vi "INIT-Settings_SERVER.vi"(7 "error in (no error)":errorcluster, 10 "Control.lvclass":refnum<class "Control-Server.lvclass">) -> (0 "error out":errorcluster, 3 "Control class out":refnum<class "Control-Server.lvclass">)   [LabVIEW 2015]
uses:
  Classes/Control/Control-Server/Control-Server.lvclass
  Classes/Config/config_names_def.ctl
  Classes/Config/Config.lvclass
  globalVarII.vi
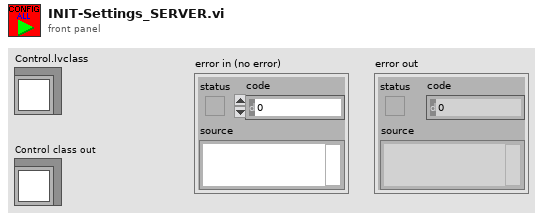
[diagram p1: front panel]
types:
  T1 = typedef "Config.lvclass/config_names_def.ctl" = string
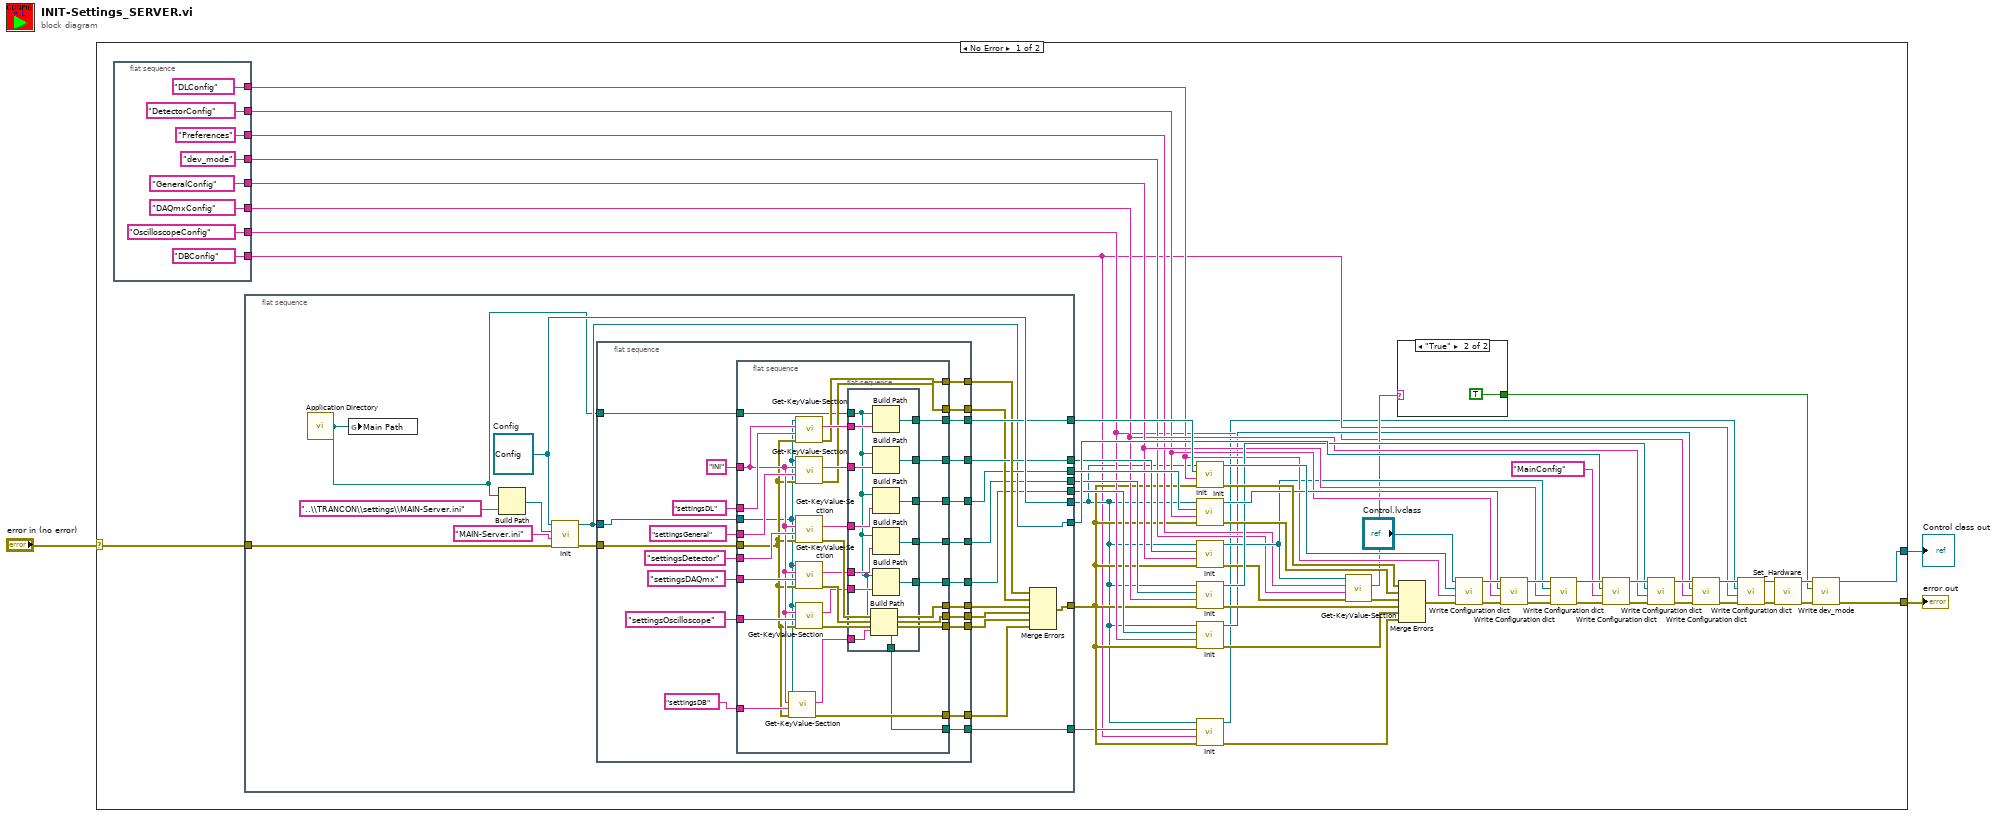
[diagram p0: block diagram]
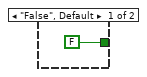
[diagram p2: hidden frame]
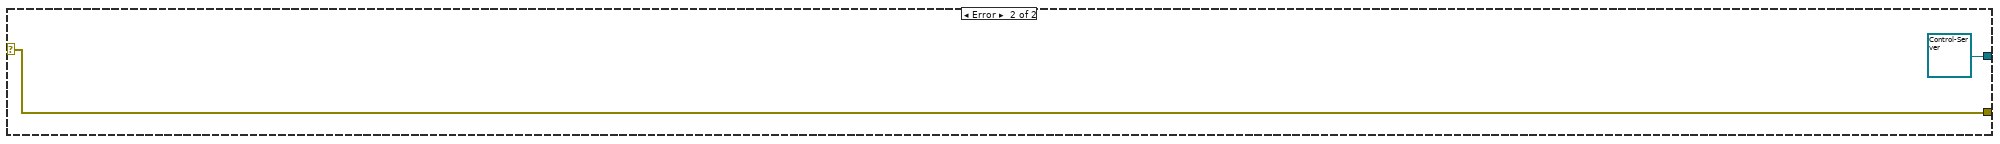
[diagram p3: hidden frame]
diagram:
  n1 = case shown="No Error" "error in (no error)" {
    selector: "error in (no error)" -> [w54 w153]
    tunnel: [w20 w153] -> w3
    tunnel: [w21 refnum<class "Control-Server.lvclass"> refnum ("Control.lvclass")] -> w1
    frame No Error {
      n2 = flat-sequence {
        tunnel: [T1 "GeneralConfig" ("Combo Box")] -> w35
        tunnel: [T1 "DAQmxConfig" ("Combo Box")] -> w34
        tunnel: [T1 "DetectorConfig" ("Combo Box")] -> w33
        tunnel: [T1 "DLConfig" ("Combo Box")] -> w32
        tunnel: ["Preferences" ("Section")] -> w25
        tunnel: ["dev_mode" ("Key")] -> w24
        tunnel: [T1 "OscilloscopeConfig" ("Combo Box")] -> w15
        tunnel: [T1 "DBConfig" ("Combo Box")] -> w5
        frame #0 {
        }
      }
      n3 = flat-sequence {
        tunnel: [w87] -> w7
        tunnel: [w84] -> w55
        tunnel: [w82] -> w39
        tunnel: w54 -> [w78]
        tunnel: [w77] -> w9
        tunnel: [w76] -> w53
        tunnel: [w75] -> w42
        tunnel: [w73] -> w38
        tunnel: [w72] -> w18
        tunnel: [w69] -> w6
        frame #0 {
          w87 = refnum<class "Config.lvclass"> refnum  # Config
          n4 = call <vilib>:"Application Directory.vi"() -> ("Application Directory"=w68:path)
          n5 = global write "globalVarII.vi" "Main Path"(w68) -> ()
          n6 = Build Path(base path=w68, name or relative path="..\\TRANCON\\settings\\MAIN-Server.ini" ("nom ou chemin relatif")) -> (appended path=w86:path)
          n7 = call "Init.vi"("error in"=w78, "Name"="MAIN-Server.ini", "Path"=w86, "Config in"=w87) -> ("error out"=w81:errorcluster, "Config out"=w75:refnum<class "Config.lvclass">)  [unwired: 6 in]
          n8 = flat-sequence {
            tunnel: [w109] -> w84
            tunnel: [w107] -> w83
            tunnel: [w106] -> w82
            tunnel: w75 -> [w105]
            tunnel: w81 -> [w102]
            tunnel: [w101] -> w80
            tunnel: [w100] -> w79
            tunnel: w68 -> [w99]
            tunnel: [w98] -> w76
            tunnel: [w96] -> w74
            tunnel: [w95] -> w73
            tunnel: [w93] -> w72
            tunnel: [w92] -> w71
            tunnel: [w90] -> w70
            tunnel: [w89] -> w69
            frame #0 {
              n9 = flat-sequence {
                tunnel: "settingsDL" ("Key") -> [w138]
                tunnel: [w136] -> w109
                tunnel: "settingsGeneral" ("Key") -> [w135]
                tunnel: [w134] -> w107
                tunnel: [w132] -> w106
                tunnel: w105 -> [w112]
                tunnel: "INI" ("Section") -> [w116]
                tunnel: "settingsDetector" ("Key") -> [w131]
                tunnel: w102 -> [w114]
                tunnel: [w130] -> w101
                tunnel: [w129] -> w100
                tunnel: w99 -> [w123]
                tunnel: [w127] -> w98
                tunnel: "settingsDAQmx" ("Key") -> [w126]
                tunnel: [w125] -> w96
                tunnel: [w122] -> w95
                tunnel: "settingsOscilloscope" ("Key") -> [w121]
                tunnel: [w119] -> w93
                tunnel: [w118] -> w92
                tunnel: "settingsDB" ("Key") -> [w117]
                tunnel: [w113] -> w90
                tunnel: [w111] -> w89
                frame #0 {
                  n10 = call-dynamic "Get-KeyValue-Section.vi"("error in (no error)"=w114, "Key"=w117, "Section"=w116, "Config in"=w112) -> ("error out"=w113:errorcluster, "Value"=w115:string)  [unwired: 5 in, 1 out]
                  n11 = call-dynamic "Get-KeyValue-Section.vi"("error in (no error)"=w114, "Key"=w138, "Section"=w116, "Config in"=w112) -> ("error out"=w134:errorcluster, "Value"=w137:string)  [unwired: 5 in, 1 out]
                  n12 = call-dynamic "Get-KeyValue-Section.vi"("error in (no error)"=w114, "Key"=w135, "Section"=w116, "Config in"=w112) -> ("error out"=w130:errorcluster, "Value"=w133:string)  [unwired: 5 in, 1 out]
                  n13 = call-dynamic "Get-KeyValue-Section.vi"("error in (no error)"=w114, "Key"=w131, "Section"=w116, "Config in"=w112) -> ("error out"=w129:errorcluster, "Value"=w128:string)  [unwired: 5 in, 1 out]
                  n14 = call-dynamic "Get-KeyValue-Section.vi"("error in (no error)"=w114, "Key"=w126, "Section"=w116, "Config in"=w112) -> ("error out"=w125:errorcluster, "Value"=w124:string)  [unwired: 5 in, 1 out]
                  n15 = call-dynamic "Get-KeyValue-Section.vi"("error in (no error)"=w114, "Key"=w121, "Section"=w116, "Config in"=w112) -> ("error out"=w118:errorcluster, "Value"=w120:string)  [unwired: 5 in, 1 out]
                  n16 = flat-sequence {
                    tunnel: w137 -> [w151]
                    tunnel: [w150] -> w136
                    tunnel: w133 -> [w149]
                    tunnel: [w148] -> w132
                    tunnel: w128 -> [w147]
                    tunnel: [w146] -> w127
                    tunnel: w124 -> [w145]
                    tunnel: w123 -> [w140]
                    tunnel: [w144] -> w122
                    tunnel: w120 -> [w143]
                    tunnel: [w142] -> w119
                    tunnel: w115 -> [w141]
                    tunnel: [w139] -> w111
                    frame #0 {
                      n17 = Build Path(base path=w140, name or relative path=w141) -> (appended path=w139:path)
                      n18 = Build Path(base path=w140, name or relative path=w151) -> (appended path=w150:path)
                      n19 = Build Path(base path=w140, name or relative path=w149) -> (appended path=w148:path)
                      n20 = Build Path(base path=w140, name or relative path=w147) -> (appended path=w146:path)
                      n21 = Build Path(base path=w140, name or relative path=w145) -> (appended path=w144:path)
                      n22 = Build Path(base path=w140, name or relative path=w143) -> (appended path=w142:path)
                    }
                  }
                }
              }
            }
          }
          n23 = Merge Errors(w83, w80, w79, w74, w71, w70) -> (w77:errorcluster)
        }
      }
      n24 = call "Init.vi"("error in"=w9, "Name"=w32, "Path"=w55, "Config in"=w7) -> ("error out"=w57:errorcluster, "Config out"=w51:refnum<class "Config.lvclass">)  [unwired: 6 in]
      n25 = call "Init.vi"("error in"=w9, "Name"=w33, "Path"=w53, "Config in"=w7) -> ("error out"=w56:errorcluster, "Config out"=w48:refnum<class "Config.lvclass">)  [unwired: 6 in]
      n26 = call "Init.vi"("error in"=w9, "Name"=w35, "Path"=w39, "Config in"=w7) -> ("error out"=w28:errorcluster, "Config out"=w26:refnum<class "Config.lvclass">)  [unwired: 6 in]
      n27 = call "Init.vi"("error in"=w9, "Name"=w34, "Path"=w38, "Config in"=w7) -> ("error out"=w36:errorcluster, "Config out"=w37:refnum<class "Config.lvclass">)  [unwired: 6 in]
      n28 = call "Init.vi"("error in"=w9, "Name"=w15, "Path"=w18, "Config in"=w7) -> ("error out"=w19:errorcluster, "Config out"=w16:refnum<class "Config.lvclass">)  [unwired: 6 in]
      n29 = call "Init.vi"("error in"=w9, "Name"=w5, "Path"=w6, "Config in"=w7) -> ("error out"=w8:errorcluster, "Config out"=w4:refnum<class "Config.lvclass">)  [unwired: 6 in]
      n30 = call-dynamic "Get-KeyValue-Section.vi"("error in (no error)"=w28, "Key"=w24, "Section"=w25, "Config in"=w26) -> ("error out"=w27:errorcluster, "Value"=w23:string)  [unwired: 5 in, 1 out]
      n31 = case shown="\"True\"" w23 {
        tunnel: [FALSE TRUE] -> w22
        frame "False", Default {
        }
        frame "True" {
        }
      }
      n32 = Merge Errors(w57, w56, w27, w36, w19, w8) -> (w46:errorcluster)
      n33 = call "Write Configuration dict.vi"("error in (no error)"=w46, "Config Name"=w32, "Config.lvclass"=w51, "Control in"="Control.lvclass") -> ("error out"=w49:errorcluster, "Control out"=w50:refnum<class "Control-Server.lvclass">)  [unwired: 6 in]
      n34 = call "Write Configuration dict.vi"("error in (no error)"=w49, "Config Name"=w33, "Config.lvclass"=w48, "Control in"=w50) -> ("error out"=w45:errorcluster, "Control out"=w47:refnum<class "Control-Server.lvclass">)  [unwired: 6 in]
      n35 = call "Write Configuration dict.vi"("error in (no error)"=w45, "Config Name"=w35, "Config.lvclass"=w26, "Control in"=w47) -> ("error out"=w44:errorcluster, "Control out"=w43:refnum<class "Control-Server.lvclass">)  [unwired: 6 in]
      n36 = call "Write Configuration dict.vi"("error in (no error)"=w44, "Config Name"=T1 "MainConfig" ("Combo Box"), "Config.lvclass"=w42, "Control in"=w43) -> ("error out"=w40:errorcluster, "Control out"=w41:refnum<class "Control-Server.lvclass">)  [unwired: 6 in]
      n37 = call "Write Configuration dict.vi"("error in (no error)"=w40, "Config Name"=w34, "Config.lvclass"=w37, "Control in"=w41) -> ("error out"=w14:errorcluster, "Control out"=w17:refnum<class "Control-Server.lvclass">)  [unwired: 6 in]
      n38 = call "Write Configuration dict.vi"("error in (no error)"=w14, "Config Name"=w15, "Config.lvclass"=w16, "Control in"=w17) -> ("error out"=w13:errorcluster, "Control out"=w10:refnum<class "Control-Server.lvclass">)  [unwired: 6 in]
      n39 = call "Write Configuration dict.vi"("error in (no error)"=w13, "Config Name"=w5, "Config.lvclass"=w4, "Control in"=w10) -> ("error out"=w12:errorcluster, "Control out"=w11:refnum<class "Control-Server.lvclass">)  [unwired: 6 in]
      n40 = call "Set_Hardware.vi"("error in (no error)"=w12, "Control in"=w11) -> ("error out"=w30:errorcluster, "Control out"=w29:refnum<class "Control-Server.lvclass">)  [unwired: 8 in]
      n41 = call-dynamic "Write dev_mode.vi"("error in (no error)"=w30, "dev_mode"=w22, "Control in"=w29) -> ("error out"=w20:errorcluster, "Control out"=w21:refnum<class "Control-Server.lvclass">)  [unwired: 7 in]
    }
    frame Error {
    }
  }
  "error out" <- w3
  "Control class out" <- w1
